vi "test call back.vi"   [LabVIEW 2017]
uses:
  D:/Software Codes/Framework/Source Code/Auto Run Screen/Source Code/IPC/MQTT/Support/MQTTdll.dll
  MQTTdll.dll
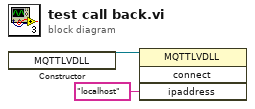
[diagram p0: block diagram]
diagram:
  n1 = constructor class="MQTTLVDLL"() -> (reference out=w2:refnum<k24>)  [unwired: 3 in, 2 out]
  n2 = invoke class="MQTTLVDLL" method="connect"(reference=w2, "ipaddress"="localhost") -> ()  [unwired: 2 in, 4 out]
